vi "故障码字段定义.vi"(7 "id":u16, 10 "首次调用？":bool, 11 "故障代码":u16(ring)) -> (3 "告警信息":T1)   [LabVIEW 2016, in "斯坦道通用流路CODmn.lvlib"]
uses:
  Alarm interface/Alarm interface.lvlib
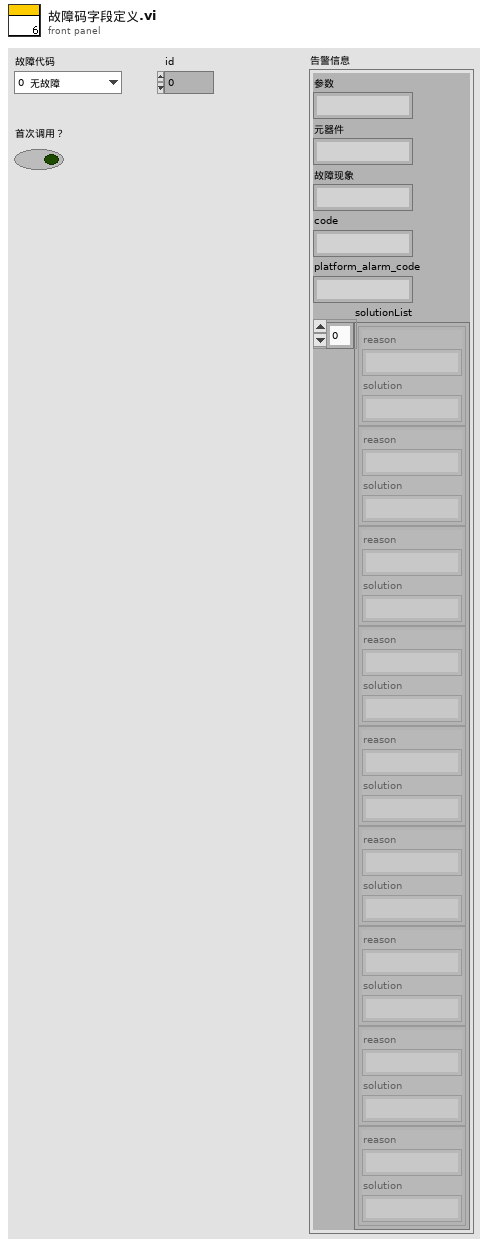
[diagram p1: front panel]
types:
  T1 = typedef "Alarm interface.lvlib/报警短信语音交互.ctl" = cluster{"参数":string, "元器件":string, "故障现象":string, "code":string, "platform_alarm_code":string, "solutionList":cluster{"reason":string, "solution":string}[]}
  T2 = cluster{"componentParent":string, "equipVersion":string, "code":string}
  T3 = typedef "SingleStepTestV3.lvlib/SingleStepTestV3.lvclass/仪器版本.ctl" = enum16{"A版", "B版", "A1版"}
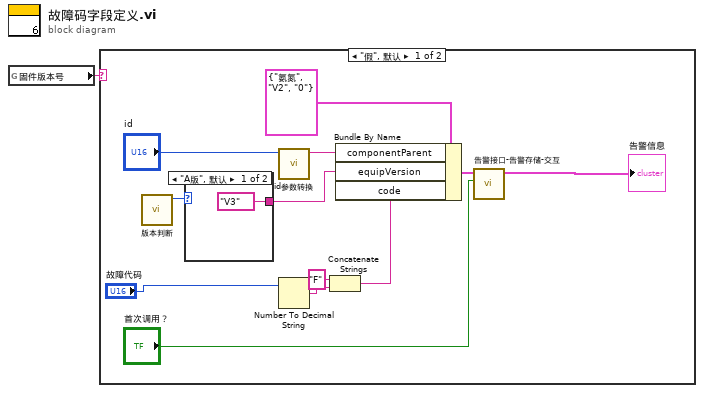
[diagram p0: block diagram]
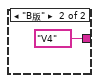
[diagram p2: hidden frame]
diagram:
  n1 = global read "VAR总磷总氮全局变量.vi" "固件版本号"() -> (w1:string)
  n2 = case shown="\"假\", 默认" w1 {
    frame "假", Default {
      n3 = call "版本判断.vi"() -> ("仪器版本"=w7:T3)  [unwired: 11 in]
      n4 = case shown="\"A版\", 默认" w7 {
        tunnel: ["V3" ("equipVersion") "V4" ("equipVersion")] -> w6
        frame "A版", Default {
        }
        frame "B版" {
        }
      }
      n5 = call "id参数转换.vi"("id"="id") -> ("table输出"=w8:string)  [unwired: 9 in, 1 out]
      n6 = Number To Decimal String(number="故障代码") -> (decimal integer string=w4:string)  [unwired: 1 in]
      n7 = Concatenate Strings("F" ("字符串"), w4) -> (w2:string)
      n8 = Bundle By Name(cluster=T2 {"componentParent"="氨氮", "equipVersion"="V2", "code"="0"} ("筛选输入"), "componentParent"=w8, "equipVersion"=w6, "code"=w2) -> (w12:T2)
      n9 = call "告警接口-告警存储-交互.vi"("首次调用？"="首次调用？", "筛选输入"=w12) -> ("data"=→"告警信息":T1)  [unwired: 9 in]
    }
    frame "" {
    }
  }
